vi "Preview Element At Index.vi"(8 "error in":errorcluster, 9 "index (-1: last)":i32=-1, 11 "Buffer in":refnum<data-value>) -> (0 "error out":errorcluster, 1 "found":bool, 2 "element":variant, 3 "Buffer":refnum<data-value>)   [LabVIEW 2013, in "VariantBuffer.lvclass"]
doc: "This VI returns data from the ring buffer starting from the oldest data and ending with the newest.\n\nThe data is duplicated at the output so this VI allocates new place in the memory for the output."
uses:
  VariantBuffer.lvclass
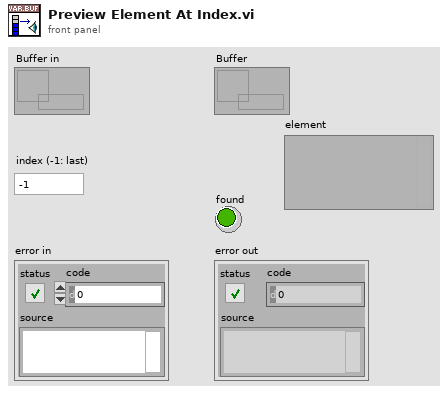
[diagram p1: front panel]
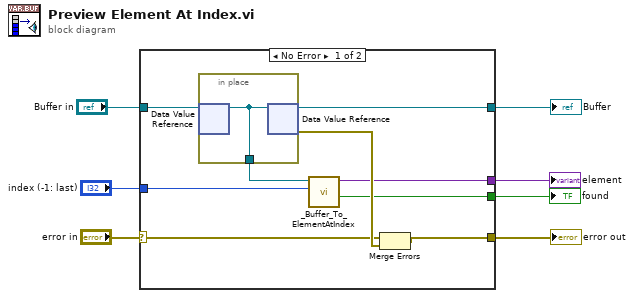
[diagram p0: block diagram]
diagram:
  n1 = case shown="No Error" "error in" {
    selector: "error in" -> [w12 w18]
    tunnel: "Buffer in" -> [w16 w19]
    tunnel: [w15 w19] -> w6
    tunnel: [w13 w18] -> w3
    tunnel: [w9 _] -> w5
    tunnel: [w8 _] -> w2
    tunnel: "index (-1: last)" -> [w10 _]
    frame No Error {
      n2 = in-place {
        in-place-border: [w17] -> w11
        n3 = in-place-dvr #1(w16) -> (w17:refnum<class "VariantBuffer.lvclass">)  [unwired: 1 out]
        n4 = in-place-dvr #1(w17) -> (w15:refnum<data-value>, w14:errorcluster)
      }
      n5 = call "_Buffer_To_ElementAtIndex.vi"("index (-1: last)"=w10, "Buffer"=w11) -> ("found"=w8:bool, "element"=w9:variant)  [unwired: 8 in]
      n6 = Merge Errors(w12, w14) -> (w13:errorcluster)
    }
    frame Error {
    }
  }
  "error out" <- w3
  "Buffer" <- w6
  "element" <- w5
  "found" <- w2
